vi "Initialize Image [Body Index].vi"(8 "error in (no error)":errorcluster) -> (0 "error out":errorcluster, 3 "Body Index Image":T1)   [LabVIEW 2014, in "LVH-KinectOne.lvlib"]
uses:
  <vilib>/vision/Image Controls.llb/IMAQ Image.ctl
  Frame Description FGV [Body Index].vi
  LVH-KinectOne.lvlib
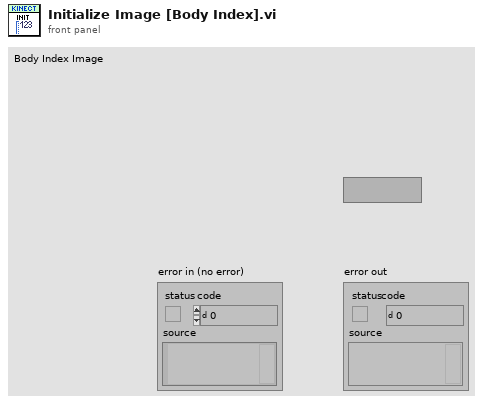
[diagram p1: front panel]
types:
  T1 = typedef "IMAQ Image.ctl" = refnum<image>
  T2 = typedef "Image Type" = u32
  T3 = typedef "LVH-KinectOne.lvlib/FrameDescription.ctl" = cluster{"BytesPerPixel":u32, "DiagonalFieldOfView":sgl, "Height":i32, "HorizontalFieldOfView":sgl, "LengthInPixels":u32, "VerticalFieldOfView":sgl, "Width":i32}
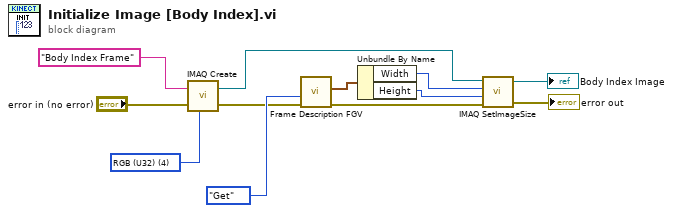
[diagram p0: block diagram]
diagram:
  w12 = T2 4 items=["Grayscale (U8)", "Grayscale (I16)", "Grayscale (SGL)", "Complex (CSG)", "RGB (U32)", "HSL (U32)", "RGB (U64)", "Grayscale (U16)"] ("Image Type")
  n1 = call "IMAQ Create"("Image Name"="Body Index Frame", "Image Type"=w12, "error in (no error)"="error in (no error)") -> ("New Image"=w3:T1, "error out"=w7:errorcluster)  [unwired: 2 in]
  n2 = call-poly "Frame Description FGV.vi"("error in (no error)"=w7, "Command"=enum16{"Get", "Set"}."Get") -> ("error out"=w6:errorcluster, "FrameDescription"=w8:T3)  [unwired: 8 in]
  n3 = Unbundle By Name(w8) -> ("Width"=w4:i32, "Height"=w5:i32)
  n4 = call "IMAQ SetImageSize"("error in (no error)"=w6, "Y Resolution"=w5, "X Resolution"=w4, "Image"=w3) -> ("error out"=→"error out":errorcluster, "Image Out"=→"Body Index Image":T1)  [unwired: 1 in]
